vi "Get Variables.vi"(8 "error in (no error)":errorcluster, 11 "Message Popup in":refnum<class "print screen.lvclass">) -> (0 "error out":errorcluster, 2 "Variables":variant, 3 "Message Popup out":refnum<class "print screen.lvclass">)   [LabVIEW 2016, in "print screen.lvclass"]
uses:
  print screen.lvclass
  print screen.lvclass/print screen.ctl
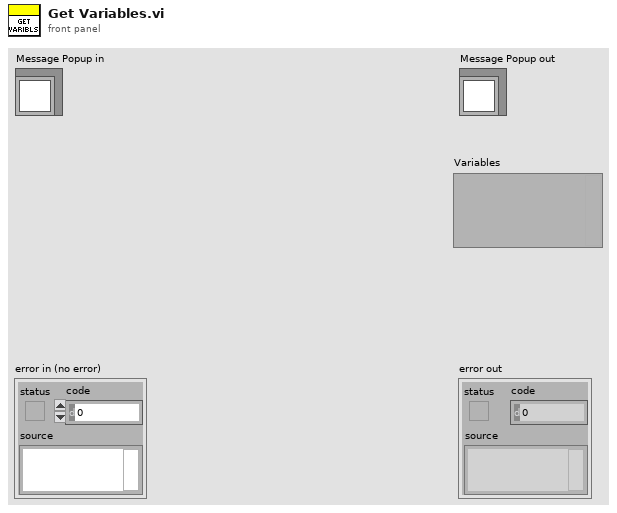
[diagram p1: front panel]
types:
  T1 = typedef "print screen.lvclass/Variables.ctl" = cluster{"message":variant}
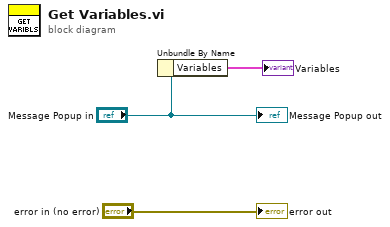
[diagram p0: block diagram]
diagram:
  n1 = Unbundle By Name("Message Popup in") -> ("Variables"=→"Variables":T1)
  "error out" <- "error in (no error)"
  "Message Popup out" <- "Message Popup in"
